vi "Get PicRedo Queue.vi"(8 "error in (no error)":errorcluster, 11 "Canvas in":refnum<class "Canvas.lvclass">) -> (0 "error out":errorcluster, 2 "PicRedo Queue":refnum<queue>, 3 "Canvas out":refnum<class "Canvas.lvclass">)   [LabVIEW 2015, in "Canvas.lvclass"]
uses:
  Canvas.lvclass
  Canvas.lvclass/Canvas.ctl
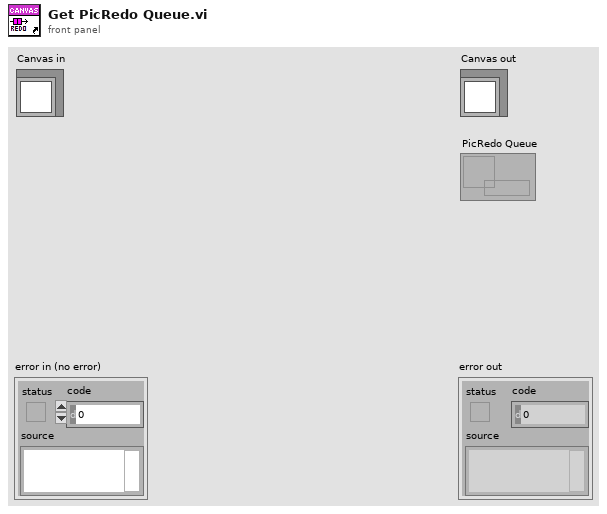
[diagram p1: front panel]
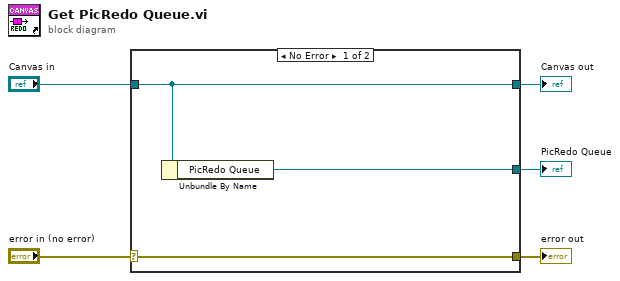
[diagram p0: block diagram]
diagram:
  n1 = case shown="No Error" "error in (no error)" {
    selector: "error in (no error)" -> [w8 w9]
    tunnel: [w8 w9] -> w4
    tunnel: [w7 w10] -> w2
    tunnel: "Canvas in" -> [w7 w10]
    tunnel: [w6 _] -> w1
    frame No Error {
      n2 = Unbundle By Name(w7) -> ("PicRedo Queue"=w6:refnum<queue>)
    }
    frame Error {
    }
  }
  "error out" <- w4
  "Canvas out" <- w2
  "PicRedo Queue" <- w1
